vi "SavePictureData.vi"(7 "File Path":path, 8 "error in (no error)":errorcluster, 9 "Exposure":u32, 10 "Index":u32, 11 "Name":string) -> (0 "error out":errorcluster)   [LabVIEW 2013]
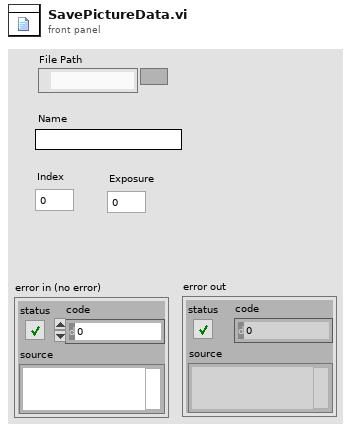
[diagram p1: front panel]
types:
  T1 = enum16{"open", "replace", "create", "open or create", "replace or create", "replace or create with confirmation"}
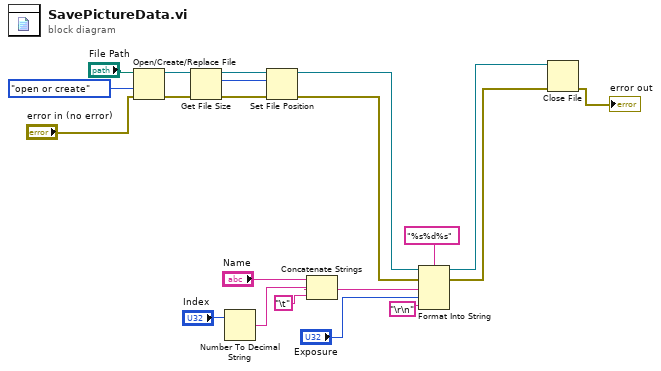
[diagram p0: block diagram]
diagram:
  n1 = Open/Create/Replace File(file path (use dialog)="File Path", error in="error in (no error)", operation (0:open)=T1."open or create") -> (refnum out=w13:refnum<file>, error out=w7:errorcluster)  [unwired: 3 in, 1 out]
  n2 = Get File Size(file=w13, error in=w7) -> (refnum out=w12:refnum<file>, size (in bytes)=w11:i64, 0:w6:errorcluster)
  n3 = Number To Decimal String(number="Index") -> (decimal integer string=w18:string)  [unwired: 1 in]
  n4 = Set File Position(offset (in bytes) (0)=w11, refnum=w12, error in=w6) -> (refnum out=w14:refnum<file>, error out=w3:errorcluster)  [unwired: 1 in]
  n5 = Concatenate Strings("Name", w18, "\t") -> (w17:string)
  n6 = Format Into String(format string="%s%d%s" ("format (%.3f)"), initial string=w14, error in=w3, w17, "Exposure", "\r\n") -> (resulting string=w20:refnum<file>, error out=w19:errorcluster)
  n7 = Close File(refnum=w20, error in=w19) -> (error out=→"error out":errorcluster)  [unwired: 1 out]
